vi "CAN 6 SPARK MAX Drivetrain Config.vi"() -> (14 "SPARK MAX Ref":T1={"FrontLeftMaster"={"DeviceStatus"={"status"=FALSE, "code"=0, "source"=""}, "Type"=enum."PWM", "PWM"={"PWM Channel"=enum."PWM 1", "DeadBand"={"Name"="", "maxPositivePwm"=0, "minPositivePwm"=0, "centerPwm"=0, "maxNegativePwm"=0, "minNegativePwm"=0, "angularRange"=0}}, "CAN"={"Device Number"=0, "SetOutput VI Ref"=variant(enum8{"Percent VBus", "Current", "Speed", "Position", "Voltage"} enum."Percent VBus"), "GetOutput VI Ref"=variant(refnum<k1> refnum), "Enable VI Ref"=variant(dbl 12.0), "Disable VI Ref"=variant(enum8{"Percent VBus", "Speed", "Position", "Slave", "Unchanged / Invalid", "Voltage Compensation", "Current", "Motion Profile"} enum."Percent VBus"), "Data"=variant}, "Invert"=FALSE, "DIO PWM"={"PWM \"Enable\" Channel"=enum."Invalid", "DIOChannel"=enum."Invalid", "PWM Rate"=0.0}}, "FrontLeftSlave1"={"DeviceStatus"={"status"=FALSE, "code"=0, "source"=""}, "Type"=enum."PWM", "PWM"={"PWM Channel"=enum."PWM 1", "DeadBand"={"Name"="", "maxPositivePwm"=0, "minPositivePwm"=0, "centerPwm"=0, "maxNegativePwm"=0, "minNegativePwm"=0, "angularRange"=0}}, "CAN"={"Device Number"=0, "SetOutput VI Ref"=variant(enum8{"Percent VBus", "Current", "Speed", "Position", "Voltage"} enum."Percent VBus"), "GetOutput VI Ref"=variant(refnum<k1> refnum), "Enable VI Ref"=variant(dbl 12.0), "Disable VI Ref"=variant(enum8{"Percent VBus", "Speed", "Position", "Slave", "Unchanged / Invalid", "Voltage Compensation", "Current", "Motion Profile"} enum."Percent VBus"), "Data"=variant}, "Invert"=FALSE, "DIO PWM"={"PWM \"Enable\" Channel"=enum."Invalid", "DIOChannel"=enum."Invalid", "PWM Rate"=0.0}}, "FrontLeftSlave2"={"DeviceStatus"={"status"=FALSE, "code"=0, "source"=""}, "Type"=enum."PWM", "PWM"={"PWM Channel"=enum."PWM 1", "DeadBand"={"Name"="", "maxPositivePwm"=0, "minPositivePwm"=0, "centerPwm"=0, "maxNegativePwm"=0, "minNegativePwm"=0, "angularRange"=0}}, "CAN"={"Device Number"=0, "SetOutput VI Ref"=variant(enum8{"Percent VBus", "Current", "Speed", "Position", "Voltage"} enum."Percent VBus"), "GetOutput VI Ref"=variant(refnum<k1> refnum), "Enable VI Ref"=variant(dbl 12.0), "Disable VI Ref"=variant(enum8{"Percent VBus", "Speed", "Position", "Slave", "Unchanged / Invalid", "Voltage Compensation", "Current", "Motion Profile"} enum."Percent VBus"), "Data"=variant}, "Invert"=FALSE, "DIO PWM"={"PWM \"Enable\" Channel"=enum."Invalid", "DIOChannel"=enum."Invalid", "PWM Rate"=0.0}}, "FrontRightMaster"={"DeviceStatus"={"status"=FALSE, "code"=0, "source"=""}, "Type"=enum."PWM", "PWM"={"PWM Channel"=enum."PWM 1", "DeadBand"={"Name"="", "maxPositivePwm"=0, "minPositivePwm"=0, "centerPwm"=0, "maxNegativePwm"=0, "minNegativePwm"=0, "angularRange"=0}}, "CAN"={"Device Number"=0, "SetOutput VI Ref"=variant(enum8{"Percent VBus", "Current", "Speed", "Position", "Voltage"} enum."Percent VBus"), "GetOutput VI Ref"=variant(refnum<k1> refnum), "Enable VI Ref"=variant(dbl 12.0), "Disable VI Ref"=variant(enum8{"Percent VBus", "Speed", "Position", "Slave", "Unchanged / Invalid", "Voltage Compensation", "Current", "Motion Profile"} enum."Percent VBus"), "Data"=variant}, "Invert"=FALSE, "DIO PWM"={"PWM \"Enable\" Channel"=enum."Invalid", "DIOChannel"=enum."Invalid", "PWM Rate"=0.0}}, "FrontRightSlave1"={"DeviceStatus"={"status"=FALSE, "code"=0, "source"=""}, "Type"=enum."PWM", "PWM"={"PWM Channel"=enum."PWM 1", "DeadBand"={"Name"="", "maxPositivePwm"=0, "minPositivePwm"=0, "centerPwm"=0, "maxNegativePwm"=0, "minNegativePwm"=0, "angularRange"=0}}, "CAN"={"Device Number"=0, "SetOutput VI Ref"=variant(enum8{"Percent VBus", "Current", "Speed", "Position", "Voltage"} enum."Percent VBus"), "GetOutput VI Ref"=variant(refnum<k1> refnum), "Enable VI Ref"=variant(dbl 12.0), "Disable VI Ref"=variant(enum8{"Percent VBus", "Speed", "Position", "Slave", "Unchanged / Invalid", "Voltage Compensation", "Current", "Motion Profile"} enum."Percent VBus"), "Data"=variant}, "Invert"=FALSE, "DIO PWM"={"PWM \"Enable\" Channel"=enum."Invalid", "DIOChannel"=enum."Invalid", "PWM Rate"=0.0}}, "FrontRightSlave2"={"DeviceStatus"={"status"=FALSE, "code"=0, "source"=""}, "Type"=enum."PWM", "PWM"={"PWM Channel"=enum."PWM 1", "DeadBand"={"Name"="", "maxPositivePwm"=0, "minPositivePwm"=0, "centerPwm"=0, "maxNegativePwm"=0, "minNegativePwm"=0, "angularRange"=0}}, "CAN"={"Device Number"=0, "SetOutput VI Ref"=variant(enum8{"Percent VBus", "Current", "Speed", "Position", "Voltage"} enum."Percent VBus"), "GetOutput VI Ref"=variant(refnum<k1> refnum), "Enable VI Ref"=variant(dbl 12.0), "Disable VI Ref"=variant(enum8{"Percent VBus", "Speed", "Position", "Slave", "Unchanged / Invalid", "Voltage Compensation", "Current", "Motion Profile"} enum."Percent VBus"), "Data"=variant}, "Invert"=FALSE, "DIO PWM"={"PWM \"Enable\" Channel"=enum."Invalid", "DIOChannel"=enum."Invalid", "PWM Rate"=0.0}}})   [LabVIEW 2018]
uses:
  SPARKMAX6Motor.ctl
  <vilib>/Rock Robotics/WPI/MotorControl/WPI_MotorControlDeviceRef.ctl
  <vilib>/Rock Robotics/WPI/MotorControl/WPI_MotorControlType.ctl
  <vilib>/Rock Robotics/SystemInterfaces/DIO/FPGA_DIOPWMChannel.ctl
  <vilib>/Rock Robotics/WPI/PWM/WPI_PWMDeadband.ctl
  <vilib>/Rock Robotics/SystemInterfaces/DIO/FPGA_DIOChannel.ctl
  <vilib>/Rock Robotics/WPI/ThirdParty/REV Robotics/SPARK MAX/Typedef/Spark MAX Status Frames.ctl
  <vilib>/Rock Robotics/WPI/ThirdParty/REV Robotics/SPARK MAX/Typedef/Spark MAX Idle Mode.ctl
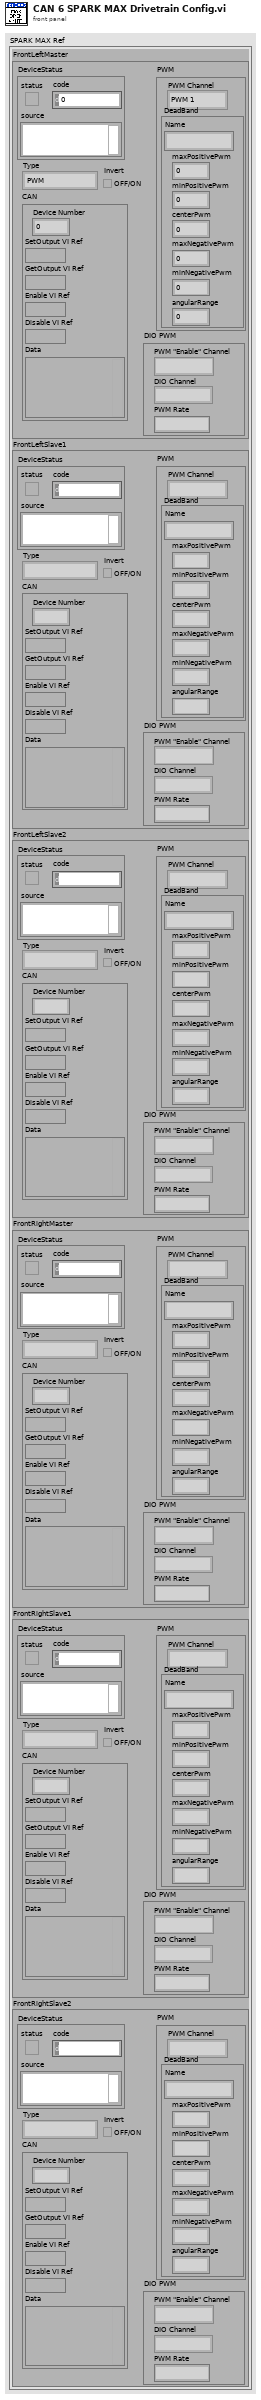
[diagram p1: front panel]
types:
  T1 = typedef "SPARKMAX6Motor.ctl" = cluster{"FrontLeftMaster":T2, "FrontLeftSlave1":T2, "FrontLeftSlave2":T2, "FrontRightMaster":T2, "FrontRightSlave1":T2, "FrontRightSlave2":T2}
  T2 = typedef "WPI_MotorControlDeviceRef.ctl" = cluster{"DeviceStatus":errorcluster, "Type":T3, "PWM":cluster{"PWM Channel":T4, "DeadBand":T5}, "CAN":cluster{"Device Number":u8, "SetOutput VI Ref":variant, "GetOutput VI Ref":variant, "Enable VI Ref":variant, "Disable VI Ref":variant, "Data":variant}, "Invert":bool, "DIO PWM":cluster{"PWM \"Enable\" Channel":T4, "DIOChannel":T6, "PWM Rate":dbl}}
  T3 = typedef "WPI_MotorControlType.ctl" = enum16{"PWM", "CAN", "DIO PWM"}
  T4 = typedef "FPGA_DIOPWMChannel.ctl" = enum8{"PWM 0", "PWM 1", "PWM 2", "PWM 3", "PWM 4", "PWM 5", "PWM 6", "PWM 7", "PWM 8", "PWM 9", "PWM MXP 0", "PWM MXP 1", "PWM MXP 2", "PWM MXP 3", "PWM MXP 4", "PWM MXP 5", "PWM MXP 6", "PWM MXP 7", "PWM MXP 8", "PWM MXP 9", "Invalid"}
  T5 = typedef "WPI_PWMDeadband.ctl" = cluster{"Name":string, "maxPositivePwm":i32, "minPositivePwm":i32, "centerPwm":i32, "maxNegativePwm":i32, "minNegativePwm":i32, "angularRange":u16}
  T6 = typedef "FPGA_DIOChannel.ctl" = enum8{"DIO 0", "DIO 1", "DIO 2", "DIO 3", "DIO 4", "DIO 5", "DIO 6", "DIO 7", "DIO 8", "DIO 9", "DIO MXP 0", "DIO MXP 1", "DIO MXP 2", "DIO MXP 3", "DIO MXP 4", "DIO MXP 5", "DIO MXP 6", "DIO MXP 7", "DIO MXP 8", "DIO MXP 9", "DIO MXP 10", "DIO MXP 11", "DIO MXP 12", "DIO MXP 13", "DIO MXP 14", "DIO MXP 15", "SPI Port CS1", "SPI Port CS2", "SPI Port CS3", "SPI Port MISO", "SPI Port MOSI", "Invalid"}
  T7 = typedef "Spark MAX Idle Mode.ctl" = enum16{"Coast", "Brake"}
  T8 = typedef "Spark MAX Status Frames.ctl" = enum16{"Status 0", "Status 1", "Status 2"}
  T9 = cluster{"P Gain":dbl, "I Gain":dbl, "D Gain":dbl, "F Gain":dbl, "I Zone":dbl, "Min Output":dbl, "Max Output":dbl}
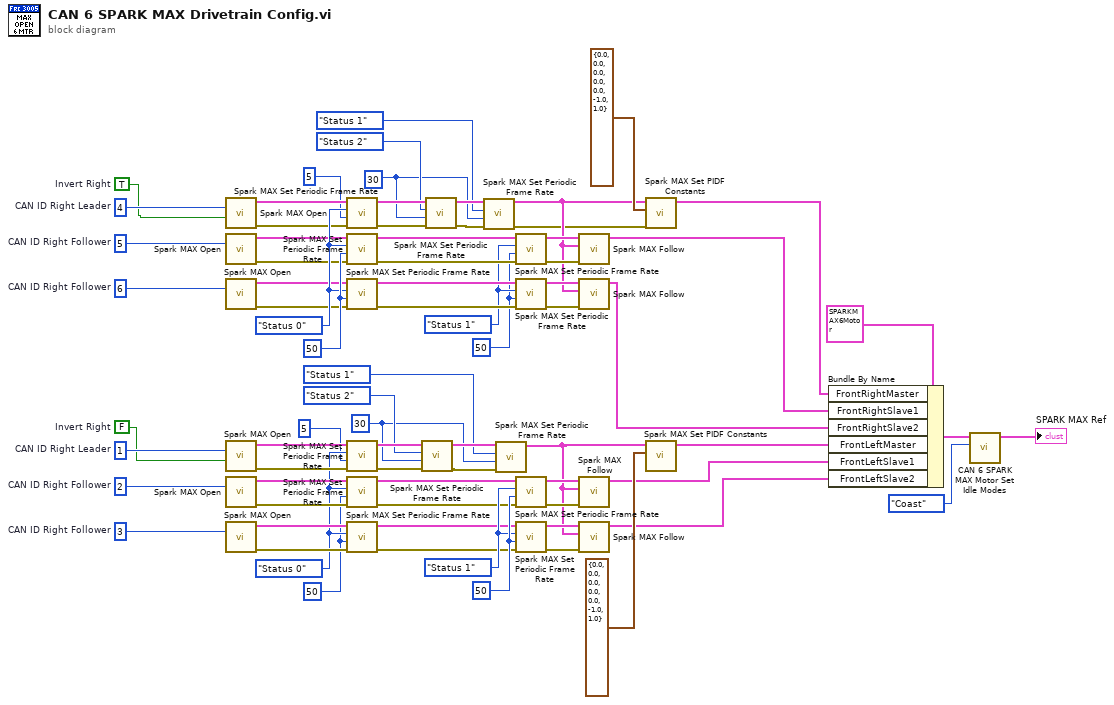
[diagram p0: block diagram]
diagram:
  w43 = u16 50 ("Frame rate (ms)")
  w44 = Spark_MAX_Status_Frames."Status 1" ("Frame")
  w42 = u16 50 ("Frame rate (ms)")
  w6 = u16 30 ("Frame rate (ms)")
  w41 = Spark_MAX_Status_Frames."Status 0" ("Frame")
  w34 = u8 6  # CAN ID Right Follower
  w8 = TRUE  # Invert Right
  w32 = u8 4  # CAN ID Right Leader
  w33 = u8 5  # CAN ID Right Follower
  w64 = u16 50 ("Frame rate (ms)")
  w63 = Spark_MAX_Status_Frames."Status 1" ("Frame")
  w65 = u16 50 ("Frame rate (ms)")
  w9 = u16 30 ("Frame rate (ms)")
  w66 = Spark_MAX_Status_Frames."Status 0" ("Frame")
  w73 = u8 3  # CAN ID Right Follower
  w7 = FALSE  # Invert Right
  w75 = u8 1  # CAN ID Right Leader
  w74 = u8 2  # CAN ID Right Follower
  n1 = call <vilib>:"Spark MAX Open.vi"("Invert"=w8, "Device Number"=w32) -> ("error out"=w40:errorcluster, "MotorControlDeviceRef"=w39:T2)  [unwired: 8 in]
  n2 = call <vilib>:"Spark MAX Open.vi"("Device Number"=w33) -> ("error out"=w37:errorcluster, "MotorControlDeviceRef"=w38:T2)  [unwired: 9 in]
  n3 = call <vilib>:"Spark MAX Open.vi"("Device Number"=w34) -> ("error out"=w35:errorcluster, "MotorControlDeviceRef"=w36:T2)  [unwired: 9 in]
  n4 = call <vilib>:"Spark MAX Open.vi"("Invert"=w7, "Device Number"=w75) -> ("error out"=w67:errorcluster, "MotorControlDeviceRef"=w68:T2)  [unwired: 8 in]
  n5 = call <vilib>:"Spark MAX Open.vi"("Device Number"=w74) -> ("error out"=w70:errorcluster, "MotorControlDeviceRef"=w69:T2)  [unwired: 9 in]
  n6 = call <vilib>:"Spark MAX Open.vi"("Device Number"=w73) -> ("error out"=w72:errorcluster, "MotorControlDeviceRef"=w71:T2)  [unwired: 9 in]
  n7 = call <vilib>:"Spark MAX Set Periodic Frame Rate.vi"("error in"=w40, "Frame rate (ms)"=u16 5, "Frame"=w41, "MotorControlDeviceRef"=w39) -> ("error out"=w24:errorcluster, "MotorControlDeviceRef"=w23:T2)  [unwired: 6 in]
  n8 = call <vilib>:"Spark MAX Set Periodic Frame Rate.vi"("error in"=w37, "Frame rate (ms)"=w42, "Frame"=w41, "MotorControlDeviceRef"=w38) -> ("error out"=w48:errorcluster, "MotorControlDeviceRef"=w45:T2)  [unwired: 6 in]
  n9 = call <vilib>:"Spark MAX Set Periodic Frame Rate.vi"("error in"=w35, "Frame rate (ms)"=w42, "Frame"=w41, "MotorControlDeviceRef"=w36) -> ("error out"=w47:errorcluster, "MotorControlDeviceRef"=w46:T2)  [unwired: 6 in]
  n10 = call <vilib>:"Spark MAX Set Periodic Frame Rate.vi"("error in"=w67, "Frame rate (ms)"=u16 5, "Frame"=w66, "MotorControlDeviceRef"=w68) -> ("error out"=w13:errorcluster, "MotorControlDeviceRef"=w14:T2)  [unwired: 6 in]
  n11 = call <vilib>:"Spark MAX Set Periodic Frame Rate.vi"("error in"=w70, "Frame rate (ms)"=w65, "Frame"=w66, "MotorControlDeviceRef"=w69) -> ("error out"=w59:errorcluster, "MotorControlDeviceRef"=w62:T2)  [unwired: 6 in]
  n12 = call <vilib>:"Spark MAX Set Periodic Frame Rate.vi"("error in"=w72, "Frame rate (ms)"=w65, "Frame"=w66, "MotorControlDeviceRef"=w71) -> ("error out"=w60:errorcluster, "MotorControlDeviceRef"=w61:T2)  [unwired: 6 in]
  n13 = call <vilib>:"Spark MAX Set Periodic Frame Rate.vi"("error in"=w13, "Frame rate (ms)"=w9, "Frame"=Spark_MAX_Status_Frames."Status 2", "MotorControlDeviceRef"=w14) -> ("error out"=w16:errorcluster, "MotorControlDeviceRef"=w15:T2)  [unwired: 6 in]
  n14 = call <vilib>:"Spark MAX Set Periodic Frame Rate.vi"("error in"=w24, "Frame rate (ms)"=w6, "Frame"=Spark_MAX_Status_Frames."Status 2", "MotorControlDeviceRef"=w23) -> ("error out"=w21:errorcluster, "MotorControlDeviceRef"=w22:T2)  [unwired: 6 in]
  n15 = call <vilib>:"Spark MAX Set Periodic Frame Rate.vi"("error in"=w21, "Frame rate (ms)"=w6, "Frame"=Spark_MAX_Status_Frames."Status 1", "MotorControlDeviceRef"=w22) -> ("error out"=w17:errorcluster, "MotorControlDeviceRef"=w18:T2)  [unwired: 6 in]
  n16 = call <vilib>:"Spark MAX Set Periodic Frame Rate.vi"("error in"=w16, "Frame rate (ms)"=w9, "Frame"=Spark_MAX_Status_Frames."Status 1", "MotorControlDeviceRef"=w15) -> ("MotorControlDeviceRef"=w12:T2)  [unwired: 6 in, 1 out]
  n17 = call <vilib>:"Spark MAX Set Periodic Frame Rate.vi"("error in"=w48, "Frame rate (ms)"=w43, "Frame"=w44, "MotorControlDeviceRef"=w45) -> ("error out"=w50:errorcluster, "MotorControlDeviceRef"=w49:T2)  [unwired: 6 in]
  n18 = call <vilib>:"Spark MAX Set Periodic Frame Rate.vi"("error in"=w47, "Frame rate (ms)"=w43, "Frame"=w44, "MotorControlDeviceRef"=w46) -> ("error out"=w51:errorcluster, "MotorControlDeviceRef"=w52:T2)  [unwired: 6 in]
  n19 = call <vilib>:"Spark MAX Set Periodic Frame Rate.vi"("error in"=w59, "Frame rate (ms)"=w64, "Frame"=w63, "MotorControlDeviceRef"=w62) -> ("error out"=w57:errorcluster, "MotorControlDeviceRef"=w58:T2)  [unwired: 6 in]
  n20 = call <vilib>:"Spark MAX Set Periodic Frame Rate.vi"("error in"=w60, "Frame rate (ms)"=w64, "Frame"=w63, "MotorControlDeviceRef"=w61) -> ("error out"=w56:errorcluster, "MotorControlDeviceRef"=w55:T2)  [unwired: 6 in]
  n21 = call <vilib>:"Spark MAX Follow.vi"("error in (no error)"=w50, "Master Controller"=w18, "MotorControlDeviceRef"=w49) -> ("MotorControlDeviceRef"=w25:T2)  [unwired: 7 in, 1 out]
  n22 = call <vilib>:"Spark MAX Follow.vi"("error in (no error)"=w51, "Master Controller"=w18, "MotorControlDeviceRef"=w52) -> ("MotorControlDeviceRef"=w26:T2)  [unwired: 7 in, 1 out]
  n23 = call <vilib>:"Spark MAX Follow.vi"("error in (no error)"=w57, "Master Controller"=w12, "MotorControlDeviceRef"=w58) -> ("MotorControlDeviceRef"=w28:T2)  [unwired: 7 in, 1 out]
  n24 = call <vilib>:"Spark MAX Follow.vi"("error in (no error)"=w56, "Master Controller"=w12, "MotorControlDeviceRef"=w55) -> ("MotorControlDeviceRef"=w27:T2)  [unwired: 7 in, 1 out]
  n25 = call <vilib>:"Spark MAX Set PIDF Constants.vi"("error in"=w17, "PID Constants"=T9 {"P Gain"=0.0, "I Gain"=0.0, "D Gain"=0.0, "F Gain"=0.0, "I Zone"=0.0, "Min Output"=-1.0, "Max Output"=1.0}, "MotorControlDeviceRef"=w18) -> ("MotorControlDeviceRef"=w30:T2)  [unwired: 7 in, 1 out]
  n26 = call <vilib>:"Spark MAX Set PIDF Constants.vi"("PID Constants"=T9 {"P Gain"=0.0, "I Gain"=0.0, "D Gain"=0.0, "F Gain"=0.0, "I Zone"=0.0, "Min Output"=-1.0, "Max Output"=1.0}, "MotorControlDeviceRef"=w12) -> ("MotorControlDeviceRef"=w29:T2)  [unwired: 8 in, 1 out]
  n27 = Bundle By Name(cluster=T1 {"FrontLeftMaster"={"DeviceStatus"={"status"=FALSE, "code"=0, "source"=""}, "Type"=enum."PWM", "PWM"={"PWM Channel"=enum."PWM 1", "DeadBand"={"Name"="", "maxPositivePwm"=0, "minPositivePwm"=0, "centerPwm"=0, "maxNegativePwm"=0, "minNegativePwm"=0, "angularRange"=0}}, "CAN"={"Device Number"=0, "SetOutput VI Ref"=variant(enum8{"Percent VBus", "Current", "Speed", "Position", "Voltage"} enum."Percent VBus"), "GetOutput VI Ref"=variant(refnum<k1> refnum), "Enable VI Ref"=variant(dbl 12.0), "Disable VI Ref"=variant(enum8{"Percent VBus", "Speed", "Position", "Slave", "Unchanged / Invalid", "Voltage Compensation", "Current", "Motion Profile"} enum."Percent VBus"), "Data"=variant}, "Invert"=FALSE, "DIO PWM"={"PWM \"Enable\" Channel"=enum."Invalid", "DIOChannel"=enum."Invalid", "PWM Rate"=0.0}}, "FrontLeftSlave1"={"DeviceStatus"={"status"=FALSE, "code"=0, "source"=""}, "Type"=enum."PWM", "PWM"={"PWM Channel"=enum."PWM 1", "DeadBand"={"Name"="", "maxPositivePwm"=0, "minPositivePwm"=0, "centerPwm"=0, "maxNegativePwm"=0, "minNegativePwm"=0, "angularRange"=0}}, "CAN"={"Device Number"=0, "SetOutput VI Ref"=variant(enum8{"Percent VBus", "Current", "Speed", "Position", "Voltage"} enum."Percent VBus"), "GetOutput VI Ref"=variant(refnum<k1> refnum), "Enable VI Ref"=variant(dbl 12.0), "Disable VI Ref"=variant(enum8{"Percent VBus", "Speed", "Position", "Slave", "Unchanged / Invalid", "Voltage Compensation", "Current", "Motion Profile"} enum."Percent VBus"), "Data"=variant}, "Invert"=FALSE, "DIO PWM"={"PWM \"Enable\" Channel"=enum."Invalid", "DIOChannel"=enum."Invalid", "PWM Rate"=0.0}}, "FrontLeftSlave2"={"DeviceStatus"={"status"=FALSE, "code"=0, "source"=""}, "Type"=enum."PWM", "PWM"={"PWM Channel"=enum."PWM 1", "DeadBand"={"Name"="", "maxPositivePwm"=0, "minPositivePwm"=0, "centerPwm"=0, "maxNegativePwm"=0, "minNegativePwm"=0, "angularRange"=0}}, "CAN"={"Device Number"=0, "SetOutput VI Ref"=variant(enum8{"Percent VBus", "Current", "Speed", "Position", "Voltage"} enum."Percent VBus"), "GetOutput VI Ref"=variant(refnum<k1> refnum), "Enable VI Ref"=variant(dbl 12.0), "Disable VI Ref"=variant(enum8{"Percent VBus", "Speed", "Position", "Slave", "Unchanged / Invalid", "Voltage Compensation", "Current", "Motion Profile"} enum."Percent VBus"), "Data"=variant}, "Invert"=FALSE, "DIO PWM"={"PWM \"Enable\" Channel"=enum."Invalid", "DIOChannel"=enum."Invalid", "PWM Rate"=0.0}}, "FrontRightMaster"={"DeviceStatus"={"status"=FALSE, "code"=0, "source"=""}, "Type"=enum."PWM", "PWM"={"PWM Channel"=enum."PWM 1", "DeadBand"={"Name"="", "maxPositivePwm"=0, "minPositivePwm"=0, "centerPwm"=0, "maxNegativePwm"=0, "minNegativePwm"=0, "angularRange"=0}}, "CAN"={"Device Number"=0, "SetOutput VI Ref"=variant(enum8{"Percent VBus", "Current", "Speed", "Position", "Voltage"} enum."Percent VBus"), "GetOutput VI Ref"=variant(refnum<k1> refnum), "Enable VI Ref"=variant(dbl 12.0), "Disable VI Ref"=variant(enum8{"Percent VBus", "Speed", "Position", "Slave", "Unchanged / Invalid", "Voltage Compensation", "Current", "Motion Profile"} enum."Percent VBus"), "Data"=variant}, "Invert"=FALSE, "DIO PWM"={"PWM \"Enable\" Channel"=enum."Invalid", "DIOChannel"=enum."Invalid", "PWM Rate"=0.0}}, "FrontRightSlave1"={"DeviceStatus"={"status"=FALSE, "code"=0, "source"=""}, "Type"=enum."PWM", "PWM"={"PWM Channel"=enum."PWM 1", "DeadBand"={"Name"="", "maxPositivePwm"=0, "minPositivePwm"=0, "centerPwm"=0, "maxNegativePwm"=0, "minNegativePwm"=0, "angularRange"=0}}, "CAN"={"Device Number"=0, "SetOutput VI Ref"=variant(enum8{"Percent VBus", "Current", "Speed", "Position", "Voltage"} enum."Percent VBus"), "GetOutput VI Ref"=variant(refnum<k1> refnum), "Enable VI Ref"=variant(dbl 12.0), "Disable VI Ref"=variant(enum8{"Percent VBus", "Speed", "Position", "Slave", "Unchanged / Invalid", "Voltage Compensation", "Current", "Motion Profile"} enum."Percent VBus"), "Data"=variant}, "Invert"=FALSE, "DIO PWM"={"PWM \"Enable\" Channel"=enum."Invalid", "DIOChannel"=enum."Invalid", "PWM Rate"=0.0}}, "FrontRightSlave2"={"DeviceStatus"={"status"=FALSE, "code"=0, "source"=""}, "Type"=enum."PWM", "PWM"={"PWM Channel"=enum."PWM 1", "DeadBand"={"Name"="", "maxPositivePwm"=0, "minPositivePwm"=0, "centerPwm"=0, "maxNegativePwm"=0, "minNegativePwm"=0, "angularRange"=0}}, "CAN"={"Device Number"=0, "SetOutput VI Ref"=variant(enum8{"Percent VBus", "Current", "Speed", "Position", "Voltage"} enum."Percent VBus"), "GetOutput VI Ref"=variant(refnum<k1> refnum), "Enable VI Ref"=variant(dbl 12.0), "Disable VI Ref"=variant(enum8{"Percent VBus", "Speed", "Position", "Slave", "Unchanged / Invalid", "Voltage Compensation", "Current", "Motion Profile"} enum."Percent VBus"), "Data"=variant}, "Invert"=FALSE, "DIO PWM"={"PWM \"Enable\" Channel"=enum."Invalid", "DIOChannel"=enum."Invalid", "PWM Rate"=0.0}}} ("TalonSRX6Motor"), "FrontRightMaster"=w30, "FrontRightSlave1"=w25, "FrontRightSlave2"=w26, "FrontLeftMaster"=w29, "FrontLeftSlave1"=w28, "FrontLeftSlave2"=w27) -> (w3:T1)
  n28 = call "CAN 6 SPARK MAX Motor Set Idle Modes.vi"("Idle Mode"=Spark_MAX_Idle_Mode."Coast", "SPARK MAX ref in"=w3) -> ("SPARK MAX ref"=→"SPARK MAX Ref":T1)  [unwired: 8 in, 1 out]
